vi "Switch_Static Dig Path Gen Close.vi"(0 "Switch Handle In":refnum<k15>, 11 "error in":errorcluster) -> (15 "error out":errorcluster)   [LabVIEW 2021, in "Switch_Static Digital Path Generation.lvlib"]
doc: "Closes the NI-SWITCH session specified in the <B>Switch Handle In</B> control and releases the resource."
uses:
  Switch_Static Digital Path Generation.lvlib
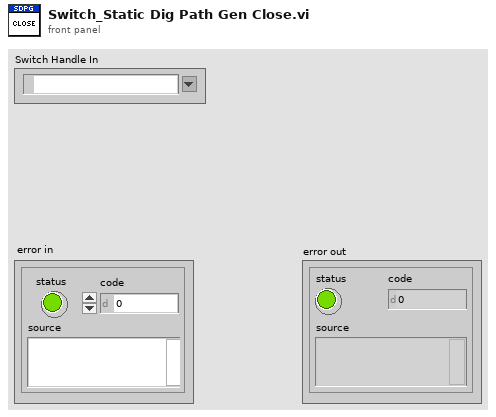
[diagram p1: front panel]
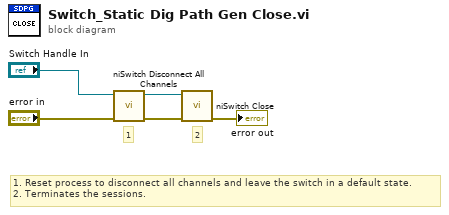
[diagram p0: block diagram]
diagram:
  # "1. Reset process to disconnect all channels and leave the switch in a default state.\n2. Terminates the sessions."
  # "2"
  # "1"
  n1 = call <instrlib>:"niSwitch Disconnect All Channels.vi"("error in (no error)"="error in", "instrument handle"="Switch Handle In") -> ("error out"=w4:errorcluster, "instrument handle out"=w5:refnum<k15>)  [unwired: 8 in]
  n2 = call <instrlib>:"niSwitch Close.vi"("error in (no error)"=w4, "instrument handle"=w5) -> ("error out"=→"error out":errorcluster)  [unwired: 9 out]
